vi "Read Dynamic Data Measurements.vi"(7 "Unit ID (A)":string="A", 8 "error in":errorcluster, 9 "Dynamic Data Info":T1, 10 "Software Rev":u8, 11 "VISA Session In":refnum<visa-resource-name>="Alicat") -> (0 "error out":errorcluster, 2 "Dynamic Data":variant[](array[variant]), 3 "VISA Session Out":refnum<visa-resource-name>)   [LabVIEW 2016]
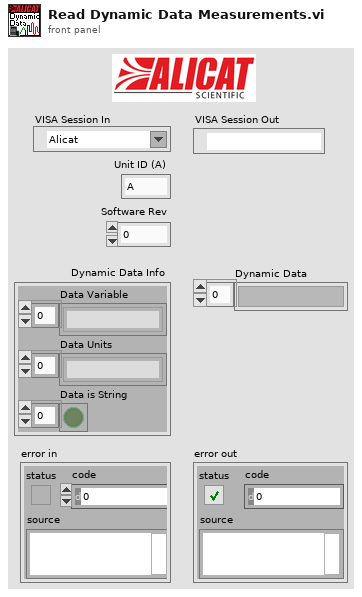
[diagram p1: front panel]
types:
  T1 = cluster{"Data Variable":string[], "Data Units":string[], "Data is String":bool[]}
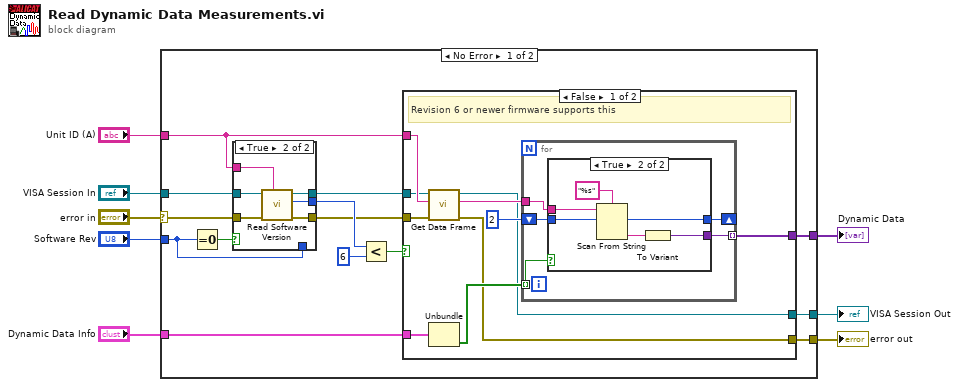
[diagram p0: block diagram]
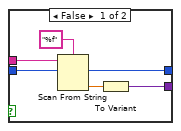
[diagram p2: hidden frame]
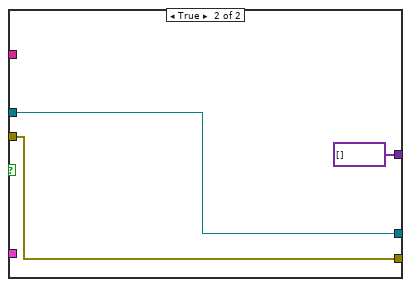
[diagram p3: hidden frame]
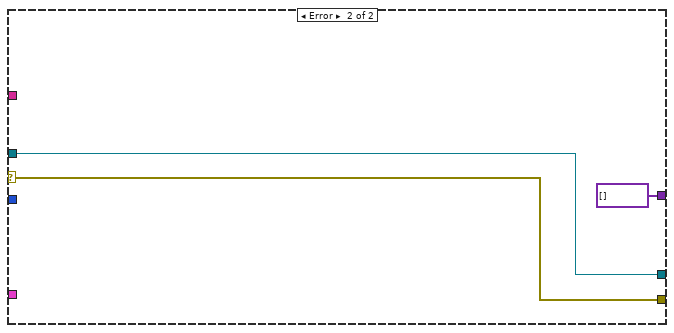
[diagram p5: hidden frame]
diagram:
  n1 = case shown="No Error" "error in" {
    selector: "error in" -> [w9 w64]
    tunnel: "VISA Session In" -> [w20 w62]
    tunnel: "Software Rev" -> [w19 _]
    tunnel: "Unit ID (A)" -> [w14 _]
    tunnel: "Dynamic Data Info" -> [w13 _]
    tunnel: [w12 variant[] []] -> w4
    tunnel: [w11 w64] -> w3
    tunnel: [w10 w62] -> w2
    frame No Error {
      n2 = Equal To 0?(x=w19) -> (x = 0?=w21:bool)
      n3 = case shown="True" w21 {
        tunnel: w9 -> [w54 w61]
        tunnel: w20 -> [w53 w60]
        tunnel: w14 -> [_ w59]
        tunnel: [w54 w58] -> w16
        tunnel: [w53 w57] -> w15
        tunnel: [w55 w56] -> w18
        tunnel: w19 -> [w55 _]
        frame False {
        }
        frame True {
          n4 = call "Read Software Version.vi"("Unit ID (A)"=w59, "error in"=w61, "VISA Session In"=w60) -> ("error out"=w58:errorcluster, "Software Version"=w56:u8, "VISA Session Out"=w57:refnum<visa-resource-name>)  [unwired: 6 in]
        }
      }
      n5 = Less?(x=w18, y=u8 6) -> (x < y?=w17:bool)
      n6 = case shown="False" w17 {
        tunnel: w16 -> [w30 w50]
        tunnel: w15 -> [w31 w51]
        tunnel: w14 -> [w32 _]
        tunnel: w13 -> [w29 _]
        tunnel: [w25 variant[] []] -> w12
        tunnel: [w24 w51] -> w10
        tunnel: [w23 w50] -> w11
        frame False {
          # "Revision 6 or newer firmware supports this"
          n7 = call "Get Data Frame.vi"("error in"=w30, "Unit ID (A)"=w32, "VISA Session In"=w31) -> ("error out"=w23:errorcluster, "Returned Data Frame"=w26:string, "VISA Session Out"=w24:refnum<visa-resource-name>)  [unwired: 6 in]
          n8 = Unbundle(w29) -> ("Data is String"=w28:bool[])  [unwired: 2 out]
          n9 = for {
            tunnel: w28 -> [w35] mode=indexing
            shift-right: [w36] -> _
            shift-left: u32 2 ("initial scan location") -> [w37]
            tunnel: [w33] -> w25 mode=indexing
            tunnel: w26 -> [w34]
            n10 = case shown="True" w35 {
              tunnel: w37 -> [w38 w49]
              tunnel: [w43 w48] -> w36
              tunnel: w34 -> [w41 w47]
              tunnel: [w39 w44] -> w33
              frame False {
                n11 = Scan From String(format string="%f", input string=w41, initial scan location=w38) -> (offset past scan=w43:u32, output 1=w40:dbl)  [unwired: 2 in, 2 out]
                n12 = To Variant(anything=w40) -> (Variant=w39:variant)
              }
              frame True {
                n13 = Scan From String(format string="%s", input string=w47, initial scan location=w49) -> (offset past scan=w48:u32, output 1=w45:string)  [unwired: 2 in, 2 out]
                n14 = To Variant(anything=w45) -> (Variant=w44:variant)
              }
            }
          }
        }
        frame True {
        }
      }
    }
    frame Error {
    }
  }
  "Dynamic Data" <- w4
  "error out" <- w3
  "VISA Session Out" <- w2
